vi "Calibration uncontrolled .vi"() -> ()   [LabVIEW 2021]
uses:
  <vilib>/MakerHub/LINX/Public/Sensors/Accelerometer/MPU60X0/DeviceAddresses.ctl
  <vilib>/MakerHub/LINX/Public/Sensors/Accelerometer/MPU60X0/GyroFullScaleRanges.ctl
  <vilib>/MakerHub/LINX/Public/Utilities/Open Serial.vi
  <vilib>/MakerHub/LINX/Public/Sensors/Motion/Servo/Servo Open One Channel.vi
  <vilib>/MakerHub/LINX/Public/Sensors/Motion/Servo/Servo Set Pulse Width One Channel.vi
  <vilib>/MakerHub/LINX/Public/Sensors/Motion/Servo/Servo Close One Channel.vi
  <vilib>/MakerHub/LINX/LMH-LINX.lvlib
  <vilib>/MakerHub/LINX/Public/Sensors/Accelerometer/MPU60X0/MPU60X0.lvlib
  <vilib>/MakerHub/LINX/Public/Sensors/Motion/Servo/Servo.lvlib
panel:
  out "Roll 2":dbl
  out "Yaw  2":dbl
  out "Pitch 2":dbl
  out "X-axis Chart 2":dbl(graph)=0.26923076923076916
  out "Z-axis Chart\n 2":dbl(graph)=0.3666666666666667
  out "Y-axis chart 2":dbl(graph)=-0.2333333333333334
  in  "stop":bool
  out "Roll Speed":dbl
  out "Pitch Speed":dbl
  out "Yaw Speed":dbl
  in  "Gyro Full Scale Range":T1=enum."±500 °/s"
  in  "Baud Rate Override":u32=115200
  in  "Serial Port":refnum<visa-resource-name>="ASRL18::INSTR"
  in  "I2C Slave Address":T2
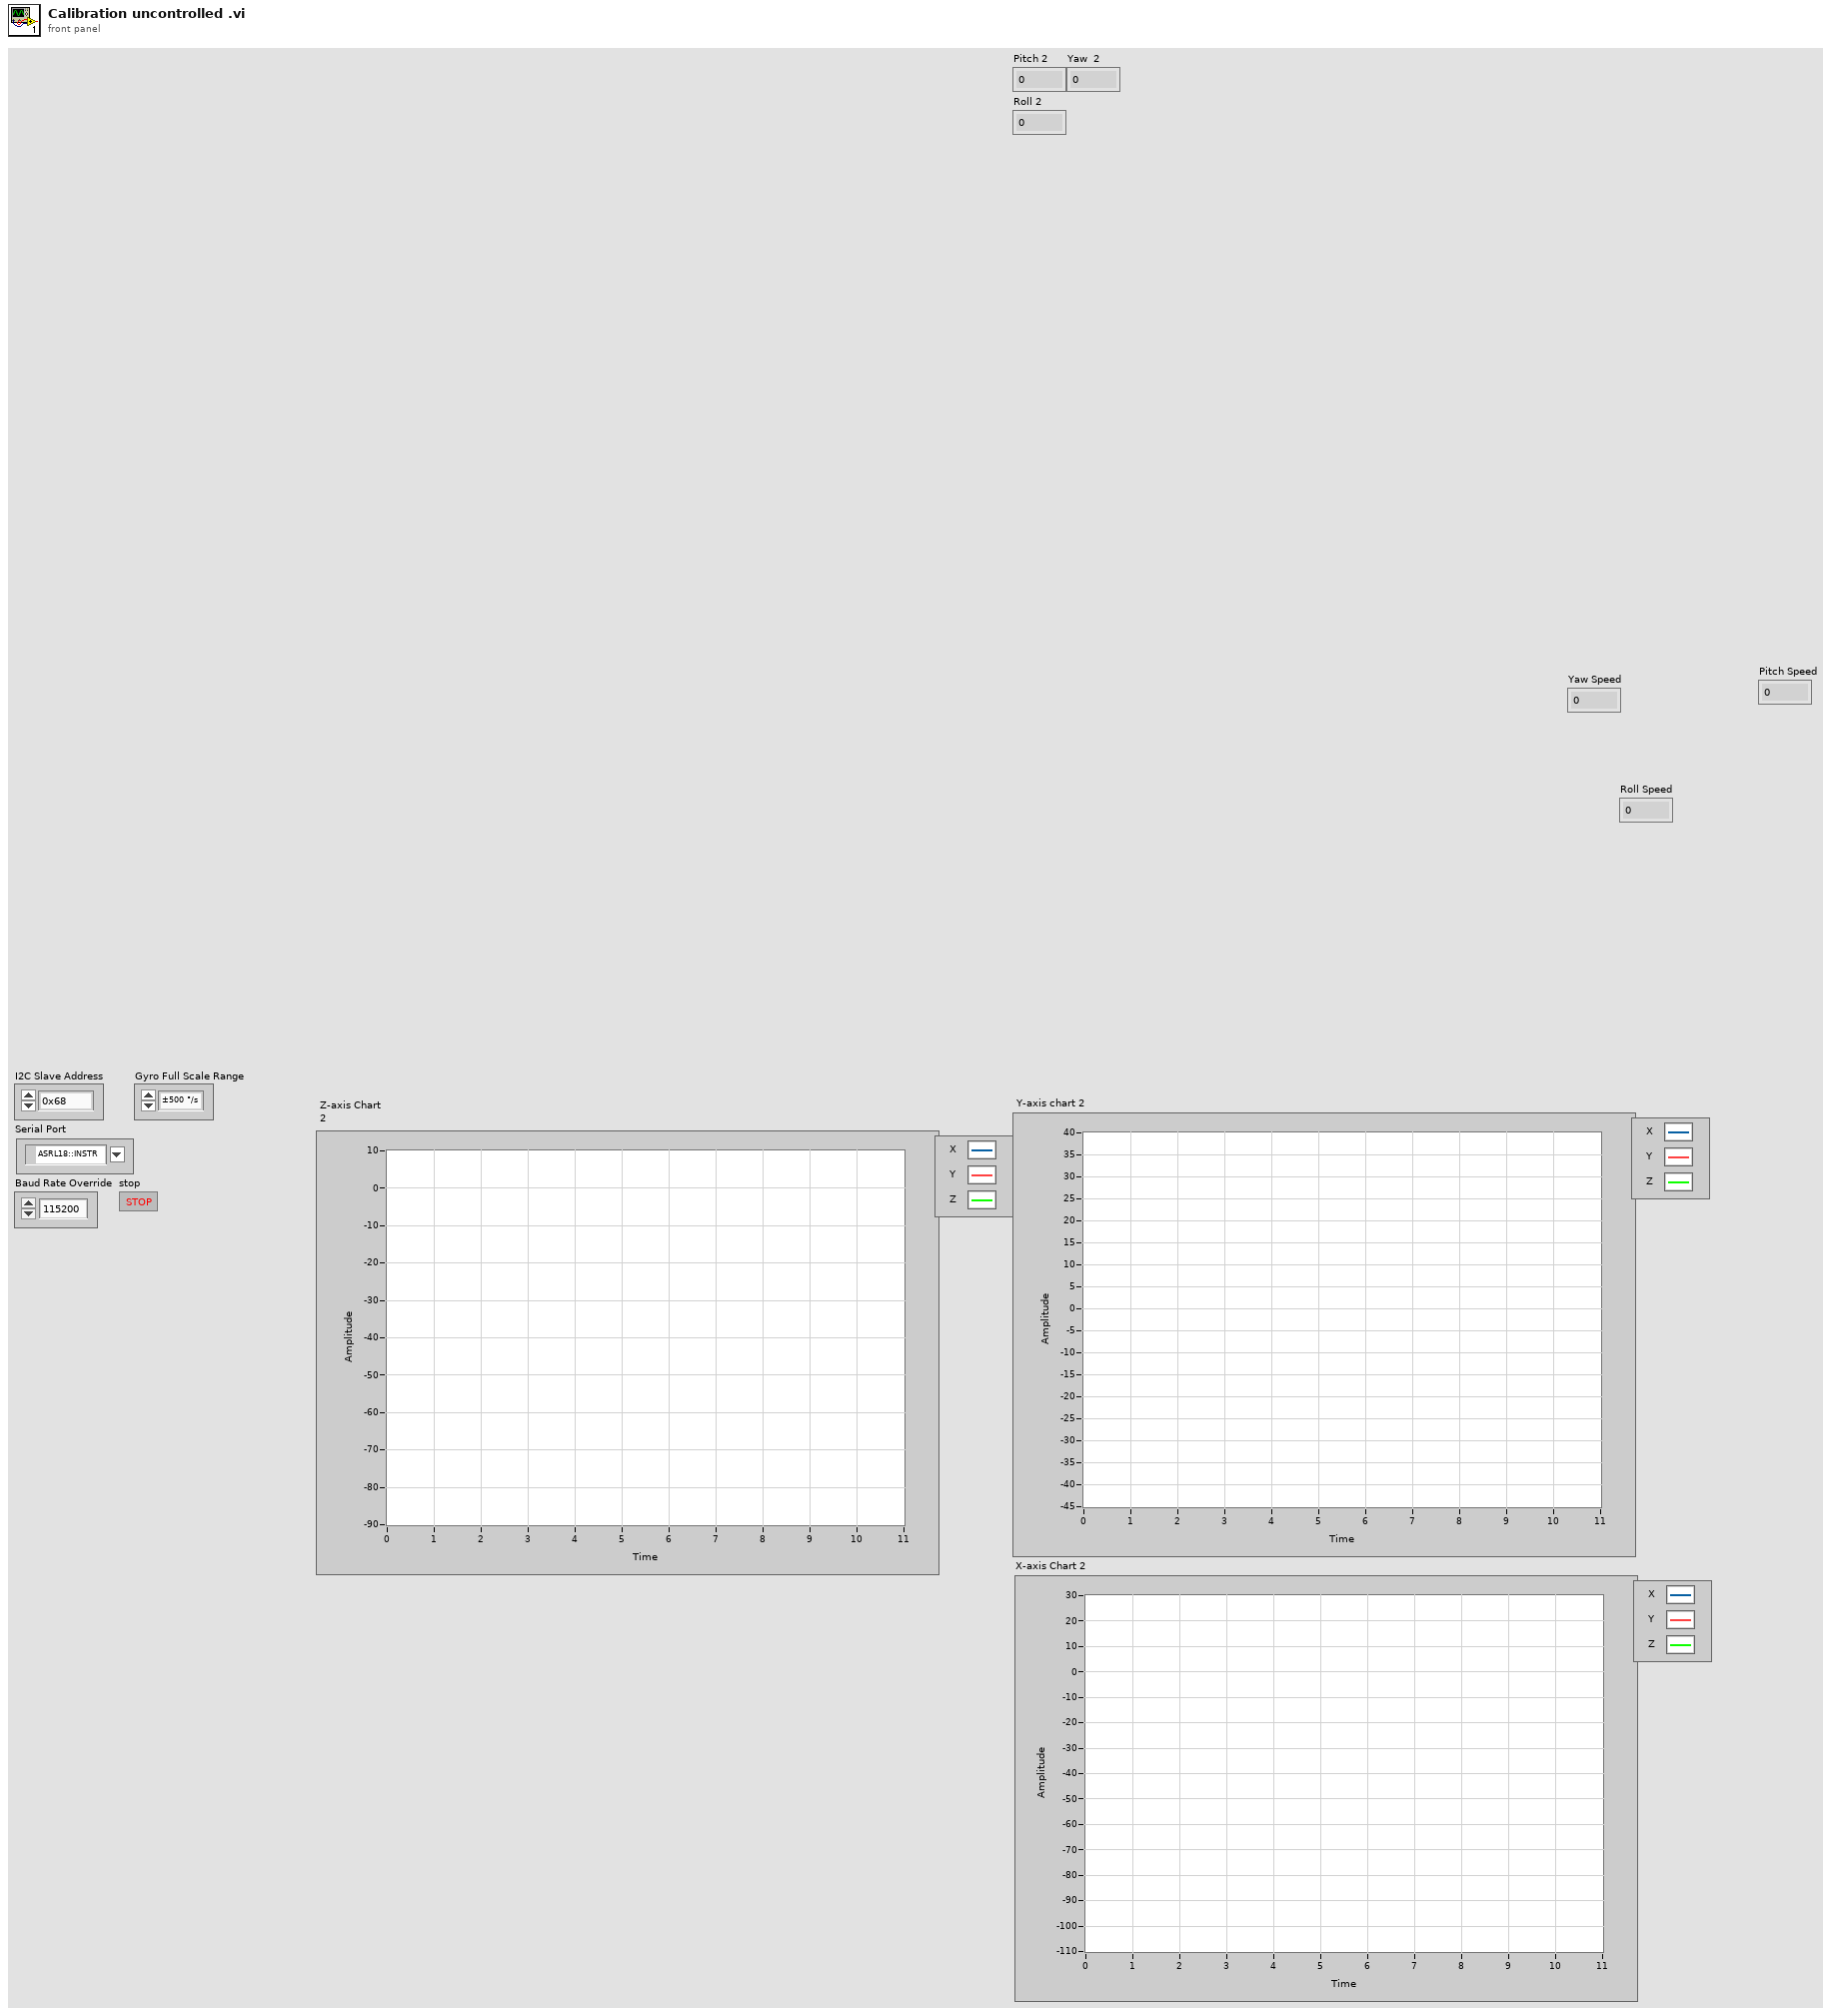
[diagram p1: front panel]
types:
  T1 = typedef "LMH-LINX.lvlib/MPU60X0.lvlib/GyroFullScaleRanges.ctl" = enum8{"±250 °/s", "±500 °/s", "±1000 °/s", "±2000 °/s"}
  T2 = typedef "LMH-LINX.lvlib/MPU60X0.lvlib/DeviceAddresses.ctl" = enum16{"0x68", "0x69"}
  T3 = typedef "LMH-LINX.lvlib/LINX Ref.ctl" = cluster{"IO":T4, "Interface":T5, "LINX Device Config":T6}
  T4 = typedef "LMH-LINX.lvlib/Platform.ctl" = enum16{"Remote", "Local"}
  T5 = typedef "LMH-LINX.lvlib/Interface.ctl" = enum16{"Serial", "TCP"}
  T6 = typedef "LMH-LINX.lvlib/Device.lvlib/LINX Device Config.ctl" = cluster{"Interface":T5, "COM Port":refnum<visa-resource-name>, "TCP Configuration":T7, "Device Family":u8, "Device ID":u8, "Device Name":string, "TCP Ref":refnum<k5>, "Channels":T8}
  T7 = typedef "LMH-LINX.lvlib/Device.lvlib/TCP Config.ctl" = cluster{"IP Address":string, "Port":u16}
  T8 = typedef "LMH-LINX.lvlib/Channels.ctl" = cluster{"DI":u8[], "DO":u8[], "AI":u8[], "AO":u8[], "PWM":u8[], "QE":u8[], "UART":u8[], "I2C 2":u8[], "SPI":u8[], "CAN":u8[], "Servo":u8[], "AI Ref (V)":dbl, "AI Resolution (Bits)":u8, "AO Ref (V)":dbl, "AO Resolution (Bits)":u8}
  T9 = cluster{"X Axis":i16, "Y Axis":i16, "Z Axis":i16}
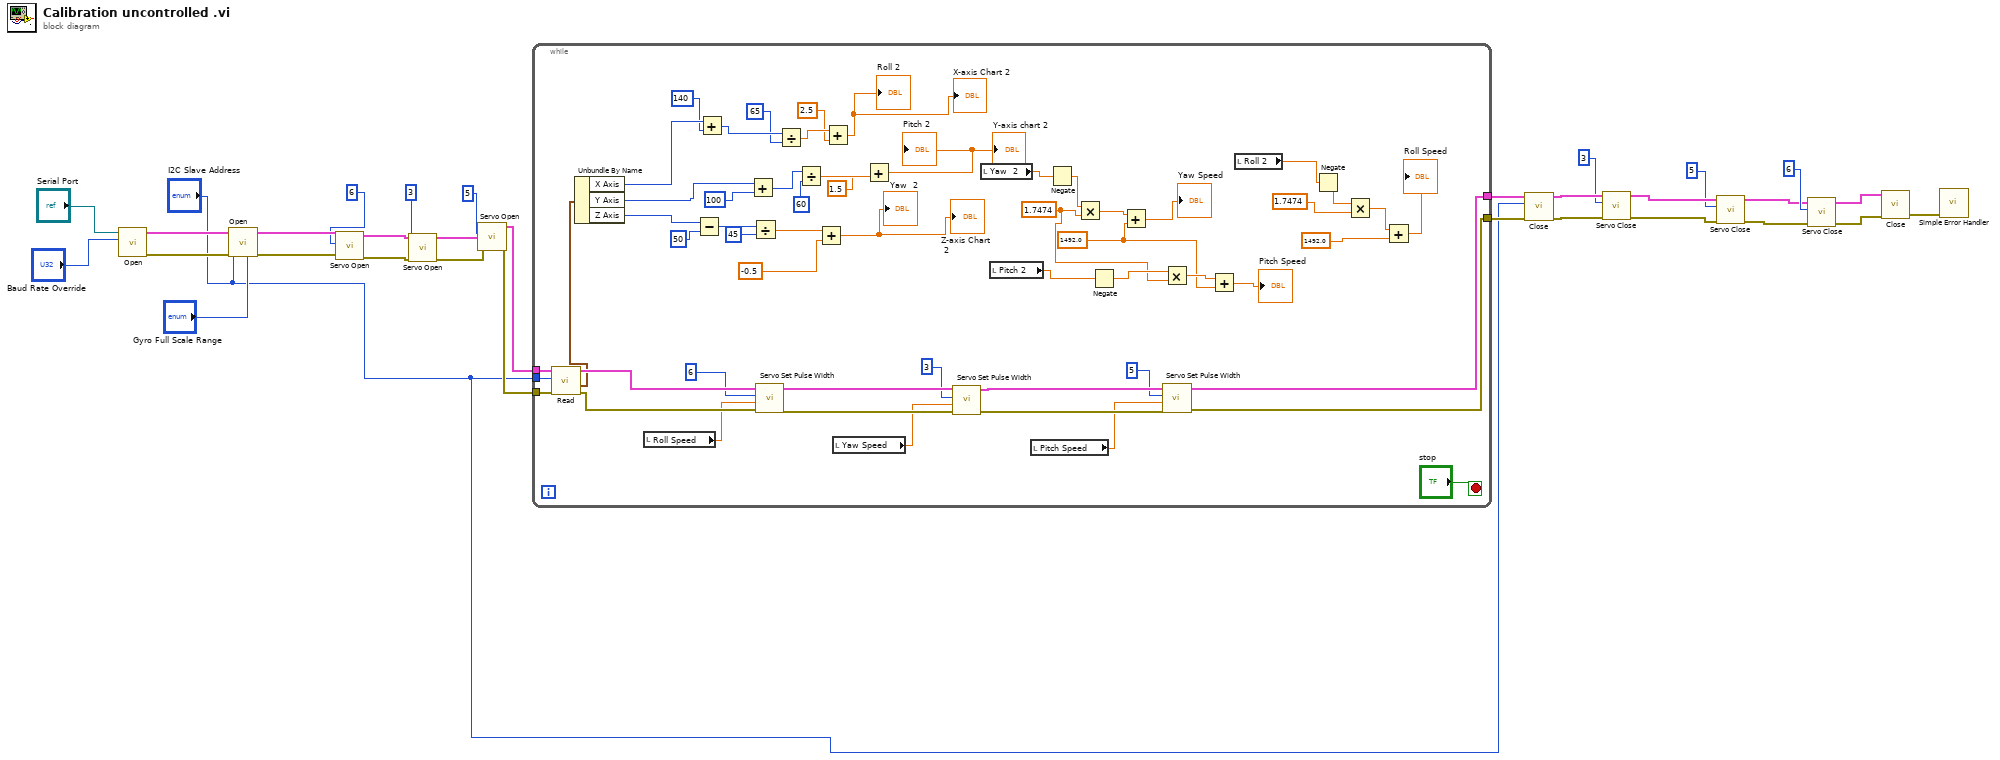
[diagram p0: block diagram]
diagram:
  n1 = call-poly <vilib>:"Open.vi"("Baud Rate Override"="Baud Rate Override", "Serial Port"="Serial Port") -> ("Error Out"=w26:errorcluster, "LINX Resource"=w27:T3)  [unwired: 7 in, 1 out]
  n2 = call <vilib>:"Open.vi"("Gyro Full Scale Range"="Gyro Full Scale Range", "Error In"=w26, "I2C Slave Address"="I2C Slave Address", "LINX Resource"=w27) -> ("Error Out"=w24:errorcluster, "LINX Resource"=w25:T3)  [unwired: 6 in]
  n3 = call-poly <vilib>:"Servo Open.vi"("Error In"=w24, "Servo Channel"=u8 6, "LINX Resource"=w25) -> ("Error Out"=w18:errorcluster, "LINX Resource"=w20:T3)  [unwired: 7 in]
  n4 = call-poly <vilib>:"Servo Open.vi"("Error In"=w18, "Servo Channel"=u8 3, "LINX Resource"=w20) -> ("Error Out"=w17:errorcluster, "LINX Resource"=w19:T3)  [unwired: 7 in]
  n5 = call-poly <vilib>:"Servo Open.vi"("Error In"=w17, "Servo Channel"=u8 5, "LINX Resource"=w19) -> ("Error Out"=w4:errorcluster, "LINX Resource"=w5:T3)  [unwired: 7 in]
  n6 = while {
    tunnel: w5 -> [w62]
    tunnel: w4 -> [w61]
    tunnel: [w60] -> w3
    tunnel: [w59] -> w2
    tunnel: "I2C Slave Address" -> [w57]
    stop <- "stop" stop-if-true
    w64 = 1.7474 ("x")
    w63 = 1492.0 ("y")
    n7 = call <vilib>:"Read.vi"("Error In"=w61, "I2C Slave Address"=w57, "LINX Resource"=w62) -> ("Error Out"=w85:errorcluster, "Gyro  Data (dps)"=w36:T9, "LINX Resource"=w86:T3)  [unwired: 4 in, 2 out]
    n8 = Unbundle By Name(w36) -> ("X Axis"=w45:i16, "Y Axis"=w53:i16, "Z Axis"=w46:i16)
    n9 = local read "Roll Speed"() -> (w74:dbl)
    n10 = Subtract(x=w46, y=i16 50) -> (x-y=w49:i16)
    n11 = Add(x=w45, y=i16 140) -> (x+y=w47:i16)
    n12 = Add(x=w53, y=i16 100) -> (x+y=w48:i16)
    n13 = Divide(x=w49, y=i16 45) -> (x/y=w52:dbl)
    n14 = call-poly <vilib>:"Servo Set Pulse Width.vi"("Error In"=w85, "Pulse Width (uS)"=w74, "Servo Channel"=u8 6, "LINX Resource"=w86) -> ("Error Out"=w78:errorcluster, "LINX Resource"=w81:T3)  [unwired: 6 in]
    n15 = Divide(x=w47, y=i16 65) -> (x/y=w50:dbl)
    n16 = Divide(x=w48, y=i16 60) -> (x/y=w51:dbl)
    n17 = Add(x=w52, y=-0.5) -> (x+y=→"Z-axis Chart\n 2" →"Yaw  2":dbl)
    n18 = Add(x=w50, y=2.5) -> (x+y=→"X-axis Chart 2" →"Roll 2":dbl)
    n19 = local read "Yaw Speed"() -> (w76:dbl)
    n20 = Add(x=w51, y=1.5) -> (x+y=→"Y-axis chart 2" →"Pitch 2":dbl)
    n21 = call-poly <vilib>:"Servo Set Pulse Width.vi"("Error In"=w78, "Pulse Width (uS)"=w76, "Servo Channel"=u8 3, "LINX Resource"=w81) -> ("Error Out"=w79:errorcluster, "LINX Resource"=w80:T3)  [unwired: 6 in]
    n22 = local read "Yaw  2"() -> (w35:dbl)
    n23 = local read "Pitch 2"() -> (w34:dbl)
    n24 = local read "Pitch Speed"() -> (w73:dbl)
    n25 = Negate(x=w35) -> (-x=w71:dbl)
    n26 = Multiply(x=w71, y=w64) -> (x*y=w87:dbl)
    n27 = Negate(x=w34) -> (-x=w69:dbl)
    n28 = Add(x=w87, y=w63) -> (x+y=→"Yaw Speed":dbl)
    n29 = Multiply(x=w69, y=w64) -> (x*y=w84:dbl)
    n30 = call-poly <vilib>:"Servo Set Pulse Width.vi"("Error In"=w79, "Pulse Width (uS)"=w73, "Servo Channel"=u8 5, "LINX Resource"=w80) -> ("Error Out"=w59:errorcluster, "LINX Resource"=w60:T3)  [unwired: 6 in]
    n31 = Add(x=w84, y=w63) -> (x+y=→"Pitch Speed":dbl)
    n32 = local read "Roll 2"() -> (w33:dbl)
    n33 = Negate(x=w33) -> (-x=w70:dbl)
    n34 = Multiply(x=w70, y=1.7474 ("x")) -> (x*y=w83:dbl)
    n35 = Add(x=w83, y=1492.0) -> (x+y=→"Roll Speed":dbl)
  }
  n36 = call <vilib>:"Close.vi"("Error In"=w2, "I2C Slave Address (0)"="I2C Slave Address", "LINX Resource"=w3) -> ("Error Out"=w10:errorcluster, "LINX Resource"=w15:T3)  [unwired: 7 in]
  n37 = call-poly <vilib>:"Servo Close.vi"("Error In"=w10, "Servo Channel"=u8 3, "LINX Resource"=w15) -> ("Error Out"=w11:errorcluster, "LINX Resource"=w14:T3)  [unwired: 7 in]
  n38 = call-poly <vilib>:"Servo Close.vi"("Error In"=w11, "Servo Channel"=u8 5, "LINX Resource"=w14) -> ("Error Out"=w12:errorcluster, "LINX Resource"=w13:T3)  [unwired: 7 in]
  n39 = call-poly <vilib>:"Servo Close.vi"("Error In"=w12, "Servo Channel"=u8 6, "LINX Resource"=w13) -> ("Error Out"=w22:errorcluster, "LINX Resource"=w21:T3)  [unwired: 7 in]
  n40 = call <vilib>:"Close.vi"("Error In"=w22, "LINX Resource"=w21) -> ("Error Out"=w31:errorcluster)  [unwired: 9 in]
  n41 = call <vilib>:"Simple Error Handler.vi"("error in (no error)"=w31) -> ()  [unwired: 4 in, 5 out]
